vi "generate array.vi"(8 "error in":errorcluster, 10 "tag bus configurable plugin module configuration":refnum<class "Tagbus PID Module configuration.lvclass">, 11 "array":T1) -> (0 "error out":errorcluster)   [LabVIEW 2014, in "Tagbus PID Module editor node.lvclass"]
uses:
  Tagbus PID Module editor node.lvclass
  PID array reference.ctl
  PID array element.ctl
  module/configuration/Tagbus PID Module configuration.lvclass
  module/configuration/PID Loop.lvclass
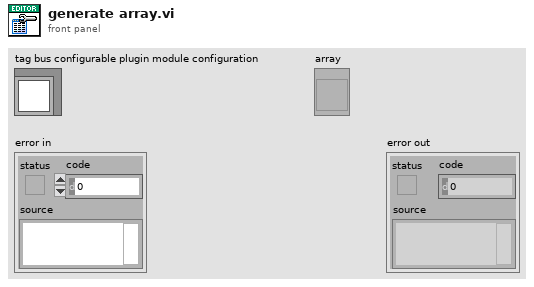
[diagram p1: front panel]
types:
  T1 = typedef "Tagbus PID Module editor node.lvclass/PID array reference.ctl" = refnum<vi>
  T2 = typedef "Tagbus PID Module editor node.lvclass/PID array element.ctl" = cluster{"Loop ID":string, "Tags":cluster{"Setpoint":string, "Process Variable":string, "Output":string}, "Gains":cluster{"P":dbl, "I":dbl, "D":dbl}, "Range":cluster{"High":dbl, "Low":dbl}}
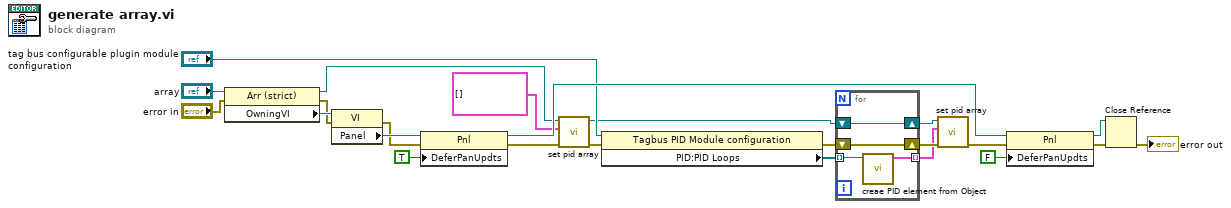
[diagram p0: block diagram]
diagram:
  n1 = property class="Arr (strict)"(reference="array", error in="error in") -> (reference out=w9:T1, error out=w14:errorcluster, "OwningVI"=w15:refnum<vi>)
  n2 = property class="VI"(reference=w15, error in=w14) -> (error out=w20:errorcluster, "Panel"=w21:refnum<vi>)  [unwired: 1 out]
  n3 = property class="Pnl"(reference=w21, error in=w20, "DeferPanUpdts"=TRUE ("Defer Panel Updates")) -> (reference out=w18:refnum<vi>, error out=w8:errorcluster)
  n4 = call "set pid array.vi"("error in (no error)"=w8, "Array"=T2[] [], "Array in"=w9) -> ("error out"=w6:errorcluster, "Array out"=w5:T1)  [unwired: 7 in]
  n5 = property class="Tagbus PID Module configuration"(reference="tag bus configurable plugin module configuration", error in=w6) -> (error out=w23:errorcluster, "PID:PID Loops"=w11:refnum<class "PID Loop.lvclass">[])  [unwired: 1 out]
  n6 = for {
    shift-right: [w25] -> w3
    shift-left: w23 -> [w25]
    shift-right: [w28] -> w4
    shift-left: w5 -> [w28]
    tunnel: w11 -> [w27] mode=indexing
    tunnel: [w26] -> w2 mode=indexing
    n7 = call "creae PID element from Object.vi"("PID Loop in"=w27) -> ("line"=w26:T2)  [unwired: 10 in]
  }
  n8 = call "set pid array.vi"("error in (no error)"=w3, "Array"=w2, "Array in"=w4) -> ("error out"=w1:errorcluster)  [unwired: 7 in, 1 out]
  n9 = property class="Pnl"(reference=w18, error in=w1, "DeferPanUpdts"=FALSE ("Defer Panel Updates")) -> (reference out=w12:refnum<vi>, error out=w17:errorcluster)
  n10 = Close Reference(reference=w12, error in (no error)=w17) -> (error out=→"error out":errorcluster)
